vi "ConvertGoop3ToGoop4_ShowBrokenVIs.vi"(0 "BrokenVIs":string[](array[string]), 1 "AppRef":refnum<vi>, 3 "ErrorsVIs":string[](array[string])) -> ()   [LabVIEW 2020]
panel:
  in  "OpenVIs":bool
  in  "Export":bool
  in  "Close":bool
  in  "Tab":T1(tab) caption="Double click to open"
  in  "Broken VIs":i32(listbox)
  in  "VIsError":i32(listbox)
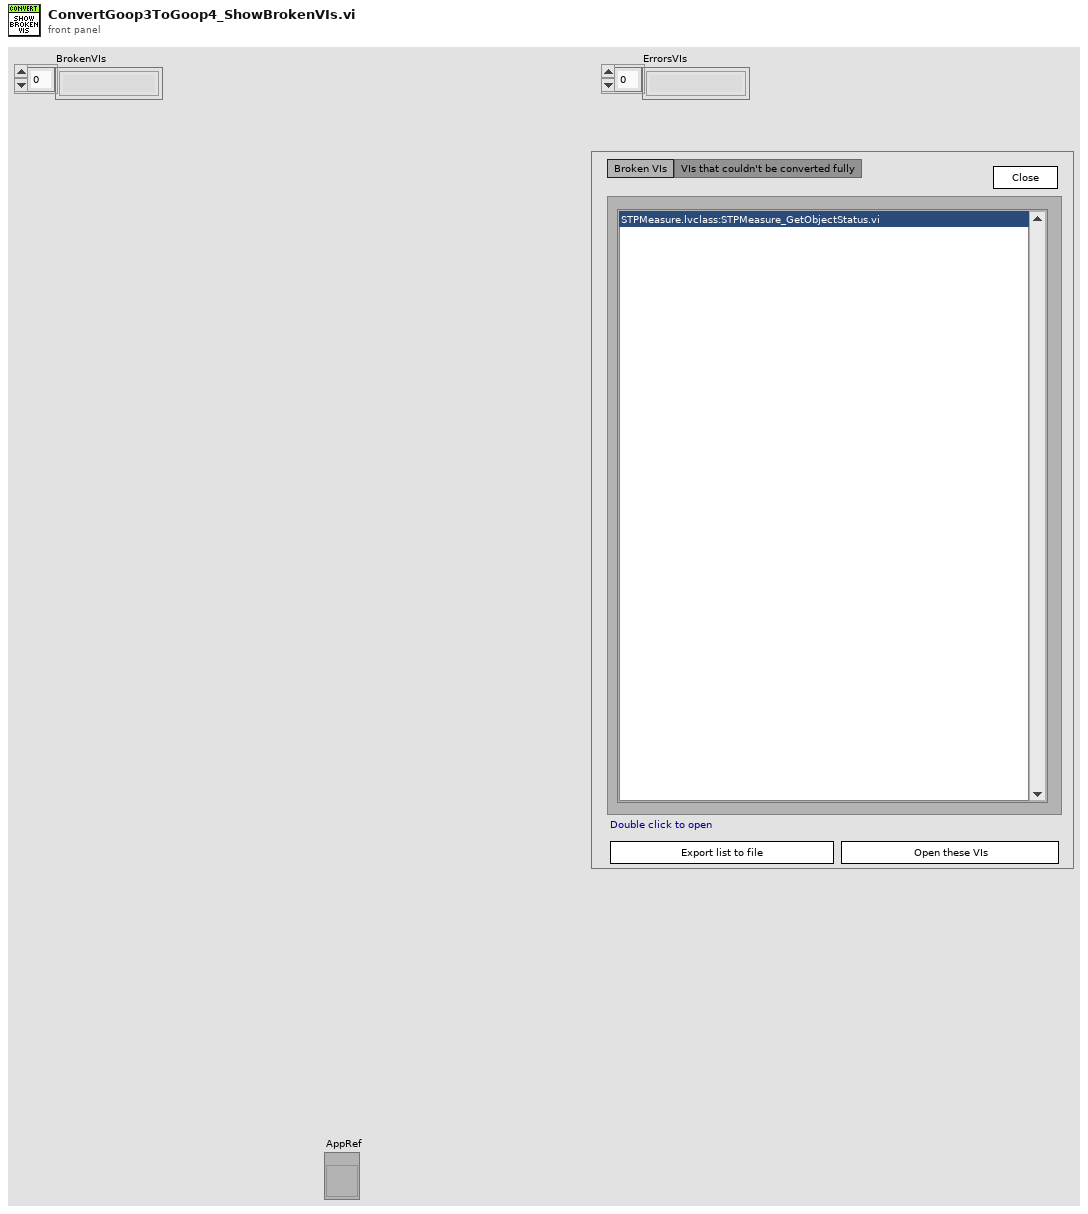
[diagram p1: front panel]
types:
  T1 = enum32{"Broken VIs", "VIs that couldn't be converted fully"}
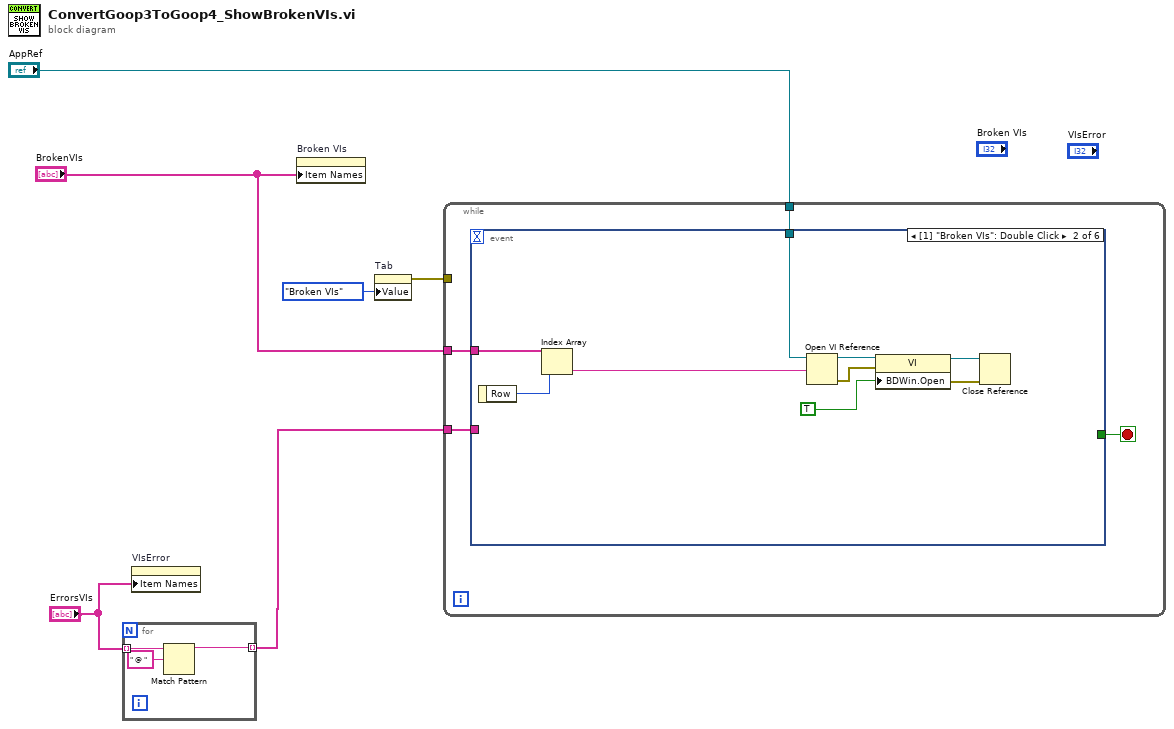
[diagram p0: block diagram]
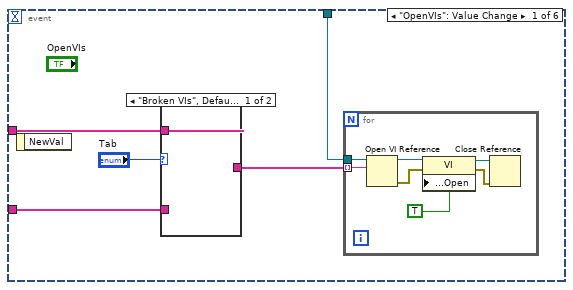
[diagram p2: hidden frame]
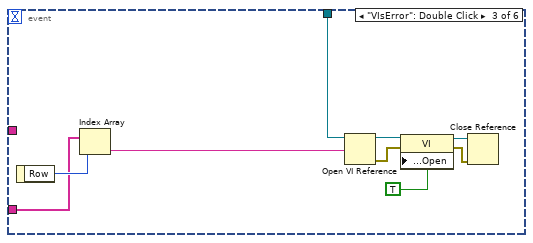
[diagram p4: hidden frame]
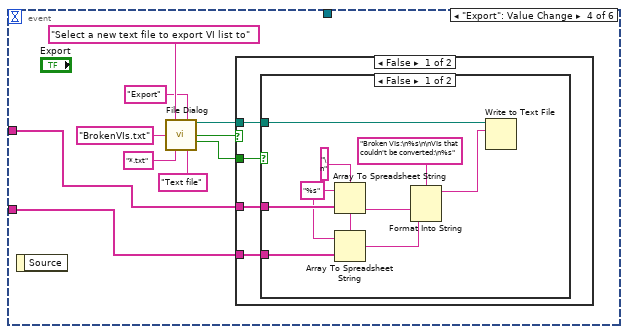
[diagram p5: hidden frame]
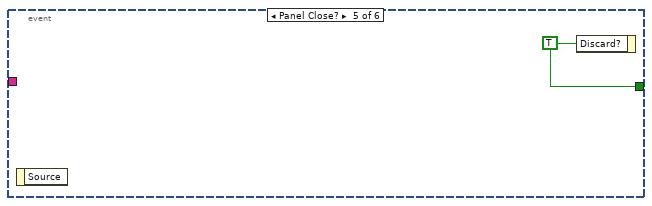
[diagram p8: hidden frame]
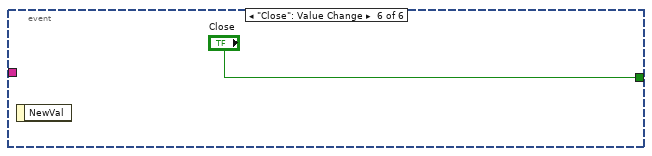
[diagram p9: hidden frame]
diagram:
  n1 = for {
    tunnel: "ErrorsVIs" -> [w9] mode=indexing
    tunnel: [w7] -> w3 mode=indexing
    n2 = Match Pattern(string=w9, regular expression=" @ ") -> (before substring=w7:string)  [unwired: 1 in, 3 out]
  }
  n3 = property on="VIsError" class="LstBox (strict)"("Item Names"="ErrorsVIs") -> ()  [unwired: 2 in, 2 out]
  n4 = property on="Broken VIs" class="LstBox (strict)"("Item Names"="BrokenVIs") -> ()  [unwired: 2 in, 2 out]
  n5 = property on="Tab" class="TabCtl (strict)"("Value"=T1."Broken VIs" ("Tab")) -> (error out=w5:errorcluster)  [unwired: 2 in, 1 out]
  n6 = while {
    tunnel: "AppRef" -> [w13]
    tunnel: "BrokenVIs" -> [w12]
    tunnel: w3 -> [w11]
    tunnel: w5 -> [_]
    stop <- w10 stop-if-true
    n7 = event shown="[1] \"Broken VIs\": Double Click" {
      selector: _ -> [_ _ _ _ _ _]
      dyn-events: _ -> [_ _ _ _ _ _]
      timeout: _ -> [_ _ _ _ _ _]
      tunnel: w13 -> [w18 w29 w38 _ _ _]
      tunnel: w12 -> [w17 w36 _ w46 _ _]
      tunnel: w11 -> [w15 _ w37 w47 _ _]
      tunnel: [_ _ _ _ w69 "Close"] -> w10
      event "OpenVIs": Value Change {
        n8 = event-data() -> ()  [unwired: 1 in, 1 out]
        n9 = case shown="\"Broken VIs\", Default" "Tab" {
          tunnel: w17 -> [w19 _]
          tunnel: [w19 w20] -> w16
          tunnel: w15 -> [_ w20]
          frame "Broken VIs", Default {
          }
          frame "VIs that couldn't be converted fully" {
          }
        }
        n10 = for {
          tunnel: w18 -> [w27]
          tunnel: w16 -> [w21] mode=indexing
          n11 = Open VI Reference(application reference (local)=w27, vi path=w21) -> (vi reference=w26:refnum<vi>, error out=w25:errorcluster)  [unwired: 4 in]
          n12 = property class="VI"(reference=w26, error in=w25, "Front Panel.Open"=TRUE ("Front Panel Window:Open")) -> (reference out=w23:refnum<vi>, error out=w22:errorcluster)
          n13 = Close Reference(reference=w23, error in (no error)=w22) -> ()  [unwired: 1 out]
        }
      }
      event "Broken VIs": Double Click {
        n14 = event-data() -> ("Row"=w35:i32)  [unwired: 1 in]
        n15 = Index Array(array=w36, index=w35) -> (element=w30:string)
        n16 = Open VI Reference(application reference (local)=w29, vi path=w30) -> (vi reference=w34:refnum<vi>, error out=w33:errorcluster)  [unwired: 4 in]
        n17 = property class="VI"(reference=w34, error in=w33, "BDWin.Open"=TRUE ("Front Panel Window:Open")) -> (reference out=w32:refnum<vi>, error out=w31:errorcluster)
        n18 = Close Reference(reference=w32, error in (no error)=w31) -> ()  [unwired: 1 out]
      }
      event "VIsError": Double Click {
        n19 = event-data() -> ("Row"=w45:i32)  [unwired: 1 in]
        n20 = Index Array(array=w37, index=w45) -> (element=w39:string)
        n21 = Open VI Reference(application reference (local)=w38, vi path=w39) -> (vi reference=w44:refnum<vi>, error out=w43:errorcluster)  [unwired: 4 in]
        n22 = property class="VI"(reference=w44, error in=w43, "Front Panel.Open"=TRUE ("Front Panel Window:Open")) -> (reference out=w41:refnum<vi>, error out=w40:errorcluster)
        n23 = Close Reference(reference=w41, error in (no error)=w40) -> ()  [unwired: 1 out]
      }
      event "Export": Value Change {
        n24 = event-data() -> ()  [unwired: 1 in, 1 out]
        n25 = call "File Dialog"("prompt"="Select a new text file to export VI list to", "button label"="Export", "default name"="BrokenVIs.txt", "pattern (all files)"="*.txt", "pattern label"="Text file") -> ("selected path"=w52:path, "exists"=w54:bool, "cancelled"=w53:bool)  [unwired: 7 in, 1 out]
        n26 = case shown="False" w54 {
          tunnel: w53 -> [w59 _]
          tunnel: w52 -> [w58 _]
          tunnel: w46 -> [w57 _]
          tunnel: w47 -> [w56 _]
          frame False {
            n27 = case shown="False" w59 {
              tunnel: w58 -> [w68 _]
              tunnel: w57 -> [w67 _]
              tunnel: w56 -> [w64 _]
              frame False {
                w65 = "%s" ("format string")
                w66 = "\n" ("delimiter (Tab)")
                n28 = Array To Spreadsheet String(delimiter (Tab)=w66, array=w67, 3:w65) -> (spreadsheet string=w63:string)
                n29 = Array To Spreadsheet String(delimiter (Tab)=w66, array=w64, 3:w65) -> (spreadsheet string=w62:string)
                n30 = Format Into String(format string="Broken VIs:\n%s\n\nVIs that couldn't be converted:\n%s", w63, w62) -> (resulting string=w60:string)  [unwired: 2 in, 1 out]
                n31 = Write to Text File(file (use dialog)=w68, text=w60) -> ()  [unwired: 2 in, 3 out]
              }
              frame True {
              }
            }
          }
          frame True {
          }
        }
      }
      event Panel Close? {
        w69 = TRUE ("Discard?")
        n32 = event-data() -> ()  [unwired: 1 in, 1 out]
        n33 = event-data("Discard?"=w69) -> ()  [unwired: 1 in, 1 out]
      }
      event "Close": Value Change {
        n34 = event-data() -> ()  [unwired: 1 in, 1 out]
      }
    }
  }
